vi "GetMindBBase.vi"(8 "错误输入（无错误）":errorcluster) -> (0 "错误输出":errorcluster, 3 "返回值":u16)   [LabVIEW 2014]
uses:
  ZXUTConfigMgr.dll
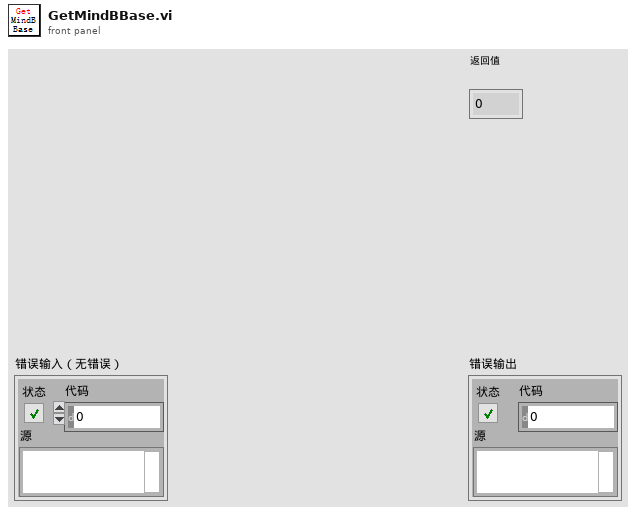
[diagram p1: front panel]
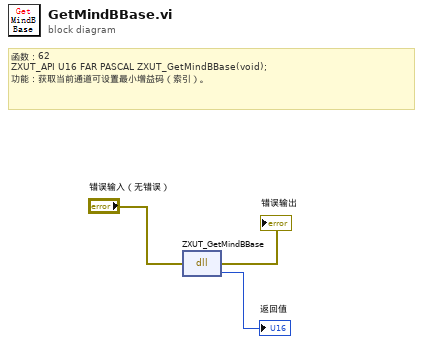
[diagram p0: block diagram]
diagram:
  # "函数：62\nZXUT_API U16\tFAR PASCAL ZXUT_GetMindBBase(void);\n功能：获取当前通道可设置最小增益码（索引）。"
  n1 = dll-call lib="PTH2eabs D软件超声实时监测软件ZXUTAppDemo(华南理工V02.00)X86DllZXUTConfigMgr.dll" fn="ZXUT_GetMindBBase"(error in="错误输入（无错误）") -> (error out=→"错误输出":errorcluster, "返回值"=→"返回值":u16)  [unwired: 2 in, 1 out]
